vi "Launcher.vi"(8 "error in (no error)":errorcluster) -> ()   [LabVIEW 2020]
uses:
  Codigo/Comunes/Controles/FGV Opciones.ctl
  Codigo/Comunes/Controles/Lista Modulos.ctl
  Codigo/Comunes/Comunicacion/Mensajes.lvlib
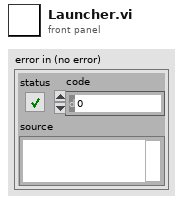
[diagram p1: front panel]
types:
  T1 = typedef "Lista Modulos.ctl" = enum16{"Math", "Error", "Front", "Database", "Nuevos items"}
  T2 = typedef "FGV Opciones.ctl" = enum16{"Get", "Create", "Destroy"}
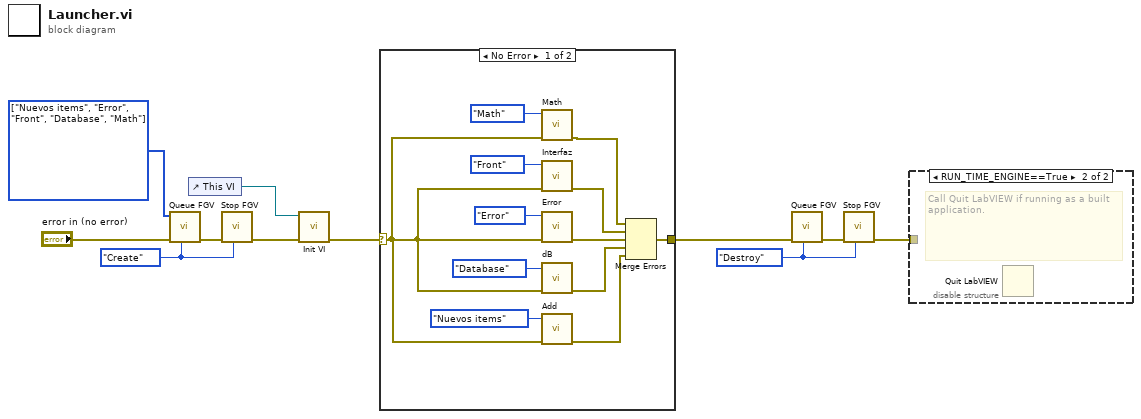
[diagram p0: block diagram]
diagram:
  w5 = T1[] [enum."Nuevos items", enum."Error", enum."Front", enum."Database", enum."Math"] items=["Math", "Error", "Front", "Database", "Nuevos items"] ("Modulos a crear")
  w7 = FGV_Opciones."Destroy" ("Enum")
  w8 = FGV_Opciones."Create" ("Enum")
  n1 = call "Queue FGV.vi"("Enum"=w8, "error in (no error)"="error in (no error)", "Modulos a crear"=w5) -> ("error out"=w11:errorcluster)  [unwired: 7 in, 1 out]
  n2 = control-ref of="This VI"() -> (w2:refnum<vi>)
  n3 = call "Stop FGV.vi"("Enum"=w8, "error in (no error)"=w11) -> ("error out"=w4:errorcluster)  [unwired: 7 in, 2 out]
  n4 = call "Init VI.vi"("error in (no error)"=w4, "VI in"=w2) -> ("error out"=w3:errorcluster)  [unwired: 9 in]
  n5 = case shown="No Error" w3 {
    selector: w3 -> [w12 w24]
    tunnel: [w22 w24] -> w6
    frame No Error {
      n6 = call "Math.vi"("error in (no error)"=w12, "Modulo a obtener"=Lista_Modulos."Math") -> ("error out"=w14:errorcluster)  [unwired: 9 in]
      n7 = call "Interfaz.vi"("error in (no error)"=w12, "Modulo a obtener"=Lista_Modulos."Front") -> ("error out"=w17:errorcluster)  [unwired: 9 in]
      n8 = call "Error.vi"("error in (no error)"=w12, "Modulo a obtener"=Lista_Modulos."Error") -> ("error out"=w23:errorcluster)  [unwired: 9 in]
      n9 = call "dB.vi"("error in (no error)"=w12, "Modulo a obtener"=Lista_Modulos."Database") -> ("error out"=w16:errorcluster)  [unwired: 9 in]
      n10 = call "Add.vi"("error in (no error)"=w12, "Modulo a obtener"=Lista_Modulos."Nuevos items") -> ("error out"=w15:errorcluster)  [unwired: 9 in]
      n11 = Merge Errors(w14, w17, w23, w16, w15) -> (w22:errorcluster)
    }
    frame Error {
    }
  }
  n12 = call "Queue FGV.vi"("Enum"=w7, "error in (no error)"=w6) -> ("error out"=w10:errorcluster)  [unwired: 8 in, 1 out]
  n13 = call "Stop FGV.vi"("Enum"=w7, "error in (no error)"=w10) -> ("error out"=w1:errorcluster)  [unwired: 7 in, 2 out]
  n14 = disable-structure shown="RUN_TIME_ENGINE==True" {
    disable-tunnel: w1 -> [_ _]
    frame condition #0 (active) {
    }
    frame condition #1 {
      # "Call Quit LabVIEW if running as a built application."
      n15 = Quit LabVIEW() -> ()  [unwired: 1 in]
    }
  }
